vi "convert_negative_blue_to_units_of_red.vi"(1 "Intensity in units of red (positive) and blue (negative)":sgl) -> (0 "Intensity in units of red (positive and negative)":sgl)   [LabVIEW 2019]
uses:
  ParametersGlobal.vi
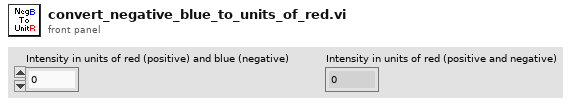
[diagram p1: front panel]
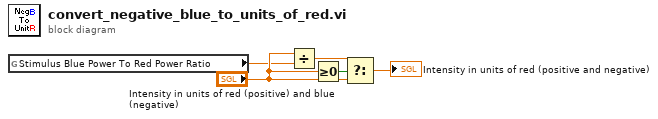
[diagram p0: block diagram]
diagram:
  n1 = global read "ParametersGlobal.vi" "Stimulus Blue Power To Red Power Ratio"() -> (w2:sgl)
  n2 = Divide(x="Intensity in units of red (positive) and blue (negative)", y=w2) -> (x/y=w3:sgl)
  n3 = Greater Or Equal To 0?(x="Intensity in units of red (positive) and blue (negative)") -> (x >= 0?=w1:bool)
  n4 = Select(t=w3, s=w1, f="Intensity in units of red (positive) and blue (negative)") -> (s? t:f=→"Intensity in units of red (positive and negative)":sgl)
